vi "rad_WriteTargetConfigOptions.vi"(8 "error in (no error)":errorcluster, 10 "TargetConfigurationOptions":T1={"NumInBatch"=0, "Target Config Operation"=enum."No Config", "Target Name"="", "Increment Static IPs"=FALSE, "Change Target Name"=FALSE, "Primary NIC"={"MAC address"="", "IP Address Request Mode"=2, "IP address"="", "Subnet mask"="", "Gateway"="", "DNS server"=""}} {"Primary NIC"."IP Address Request Mode" items=["Static"=1, "DHCP/Link-Local"=2, "Link-Local Only"=4, "DHCP Only"=8]}, 11 "configuration file path":path) -> (0 "error out":errorcluster)   [LabVIEW 2013]
uses:
  App Images/TypeDefs/rad_Target Configuration Settings.ctl
  App Images/TypeDefs/rad_Target Configuration Operations.ctl
  TypeDefs/rad_Target Network Settings.ctl
  <vilib>/Utility/config.llb/Write Key (U32).vi
  <vilib>/Utility/config.llb/Write Key (I32).vi
  <vilib>/Utility/config.llb/Write Key (String).vi
  <vilib>/Utility/config.llb/Write Key (Boolean).vi
  <vilib>/Utility/config.llb/NI_LVConfig.lvlib
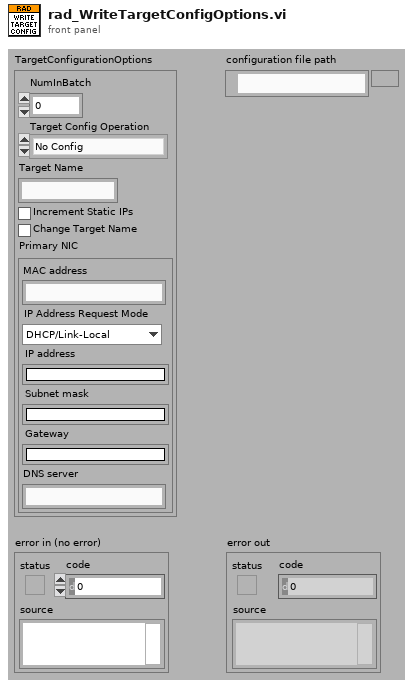
[diagram p1: front panel]
types:
  T1 = typedef "rad_Target Configuration Settings.ctl" = cluster{"NumInBatch":u32, "Target Config Operation":T2, "Target Name":string, "Increment Static IPs":bool, "Change Target Name":bool, "Primary NIC":T3}
  T2 = typedef "rad_Target Configuration Operations.ctl" = enum8{"No Config", "Image Config", "Static Config"}
  T3 = typedef "rad_Target Network Settings.ctl" = cluster{"MAC address":string, "IP Address Request Mode":i32, "IP address":string, "Subnet mask":string, "Gateway":string, "DNS server":string}
  T4 = typedef "NI_LVConfig.lvlib/Config Data RefNum.ctl" = refnum<k1>
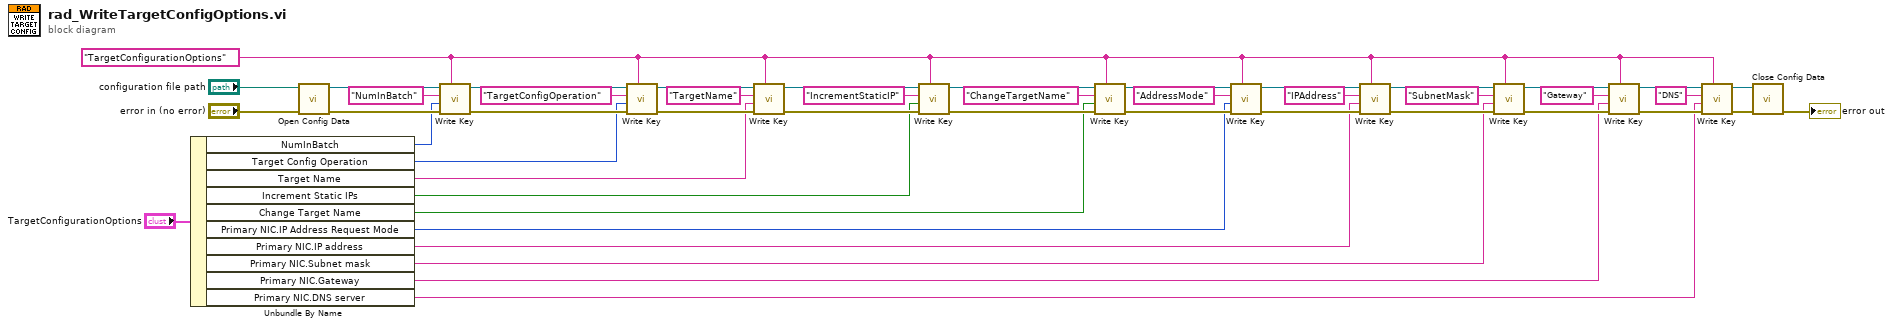
[diagram p0: block diagram]
diagram:
  w22 = "TargetConfigurationOptions" ("section")
  n1 = Unbundle By Name("TargetConfigurationOptions") -> ("NumInBatch"=w10:u32, "Target Config Operation"=w9:T2, "Target Name"=w8:string, "Increment Static IPs"=w7:bool, "Change Target Name"=w6:bool, "Primary NIC.IP Address Request Mode"=w5:i32, "Primary NIC.IP address"=w4:string, "Primary NIC.Subnet mask"=w3:string, "Primary NIC.Gateway"=w2:string, "Primary NIC.DNS server"=w1:string)
  n2 = call <vilib>:"Open Config Data.vi"("error in (no error)"="error in (no error)", "configuration file path"="configuration file path") -> ("error out"=w45:errorcluster, "refnum"=w46:T4)  [unwired: 7 in, 1 out]
  n3 = call-poly <vilib>:"Write Key.vi"("section"=w22, "error in (no error)"=w45, "value"=w10, "key"="NumInBatch", "refnum"=w46) -> ("error out"=w41:errorcluster, "refnum out"=w42:T4)  [unwired: 4 in, 1 out]
  n4 = call-poly <vilib>:"Write Key.vi"("section"=w22, "error in (no error)"=w41, "value"=w9, "key"="TargetConfigOperation", "refnum"=w42) -> ("error out"=w39:errorcluster, "refnum out"=w38:T4)  [unwired: 4 in, 1 out]
  n5 = call-poly <vilib>:"Write Key.vi"("section"=w22, "error in (no error)"=w39, "value"=w8, "key"="TargetName", "refnum"=w38) -> ("error out"=w26:errorcluster, "refnum out"=w18:T4)  [unwired: 4 in, 1 out]
  n6 = call-poly <vilib>:"Write Key.vi"("section"=w22, "error in (no error)"=w26, "value"=w7, "key"="IncrementStaticIP", "refnum"=w18) -> ("error out"=w25:errorcluster, "refnum out"=w17:T4)  [unwired: 4 in, 1 out]
  n7 = call-poly <vilib>:"Write Key.vi"("section"=w22, "error in (no error)"=w25, "value"=w6, "key"="ChangeTargetName", "refnum"=w17) -> ("error out"=w24:errorcluster, "refnum out"=w16:T4)  [unwired: 4 in, 1 out]
  n8 = call-poly <vilib>:"Write Key.vi"("section"=w22, "error in (no error)"=w24, "value"=w5, "key"="AddressMode", "refnum"=w16) -> ("error out"=w23:errorcluster, "refnum out"=w15:T4)  [unwired: 4 in, 1 out]
  n9 = call-poly <vilib>:"Write Key.vi"("section"=w22, "error in (no error)"=w23, "value"=w4, "key"="IPAddress", "refnum"=w15) -> ("error out"=w21:errorcluster, "refnum out"=w14:T4)  [unwired: 4 in, 1 out]
  n10 = call-poly <vilib>:"Write Key.vi"("section"=w22, "error in (no error)"=w21, "value"=w3, "key"="SubnetMask", "refnum"=w14) -> ("error out"=w20:errorcluster, "refnum out"=w13:T4)  [unwired: 4 in, 1 out]
  n11 = call-poly <vilib>:"Write Key.vi"("section"=w22, "error in (no error)"=w20, "value"=w2, "key"="Gateway", "refnum"=w13) -> ("error out"=w19:errorcluster, "refnum out"=w12:T4)  [unwired: 4 in, 1 out]
  n12 = call-poly <vilib>:"Write Key.vi"("section"=w22, "error in (no error)"=w19, "value"=w1, "key"="DNS", "refnum"=w12) -> ("error out"=w30:errorcluster, "refnum out"=w29:T4)  [unwired: 4 in, 1 out]
  n13 = call <vilib>:"Close Config Data.vi"("error in (no error)"=w30, "refnum"=w29) -> ("error out"=→"error out":errorcluster)  [unwired: 8 in, 1 out]
